vi "VibSystem3Signals.vi"(8 "sampling info":cluster{"Fs":dbl, "#s":dbl}={"Fs"=10000.0, "#s"=10000.0} {"Fs" format="%.2p"}, 9 "Temperature Channels Voltage In":dbl[](array[numeric]), 10 "Frequency":dbl, 11 "Constant Amplitudes?":bool) -> (1 "Temperature Channels Voltage Out":dbl[](array[numeric]), 3 "Signals":waveform(dbl)[](array[waveform]))   [LabVIEW 2017]
uses:
  <vilib>/measure/NI_MABase.lvlib
panel:
  out "Waveform Graph":waveform(dbl)[](graph)
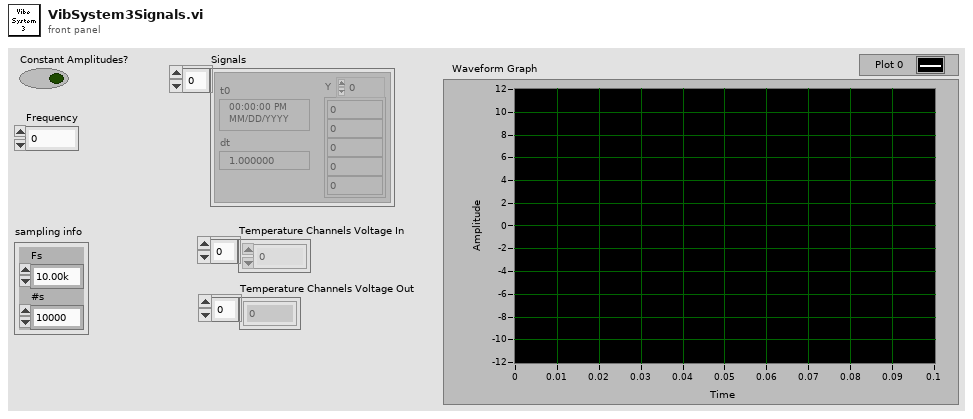
[diagram p1: front panel]
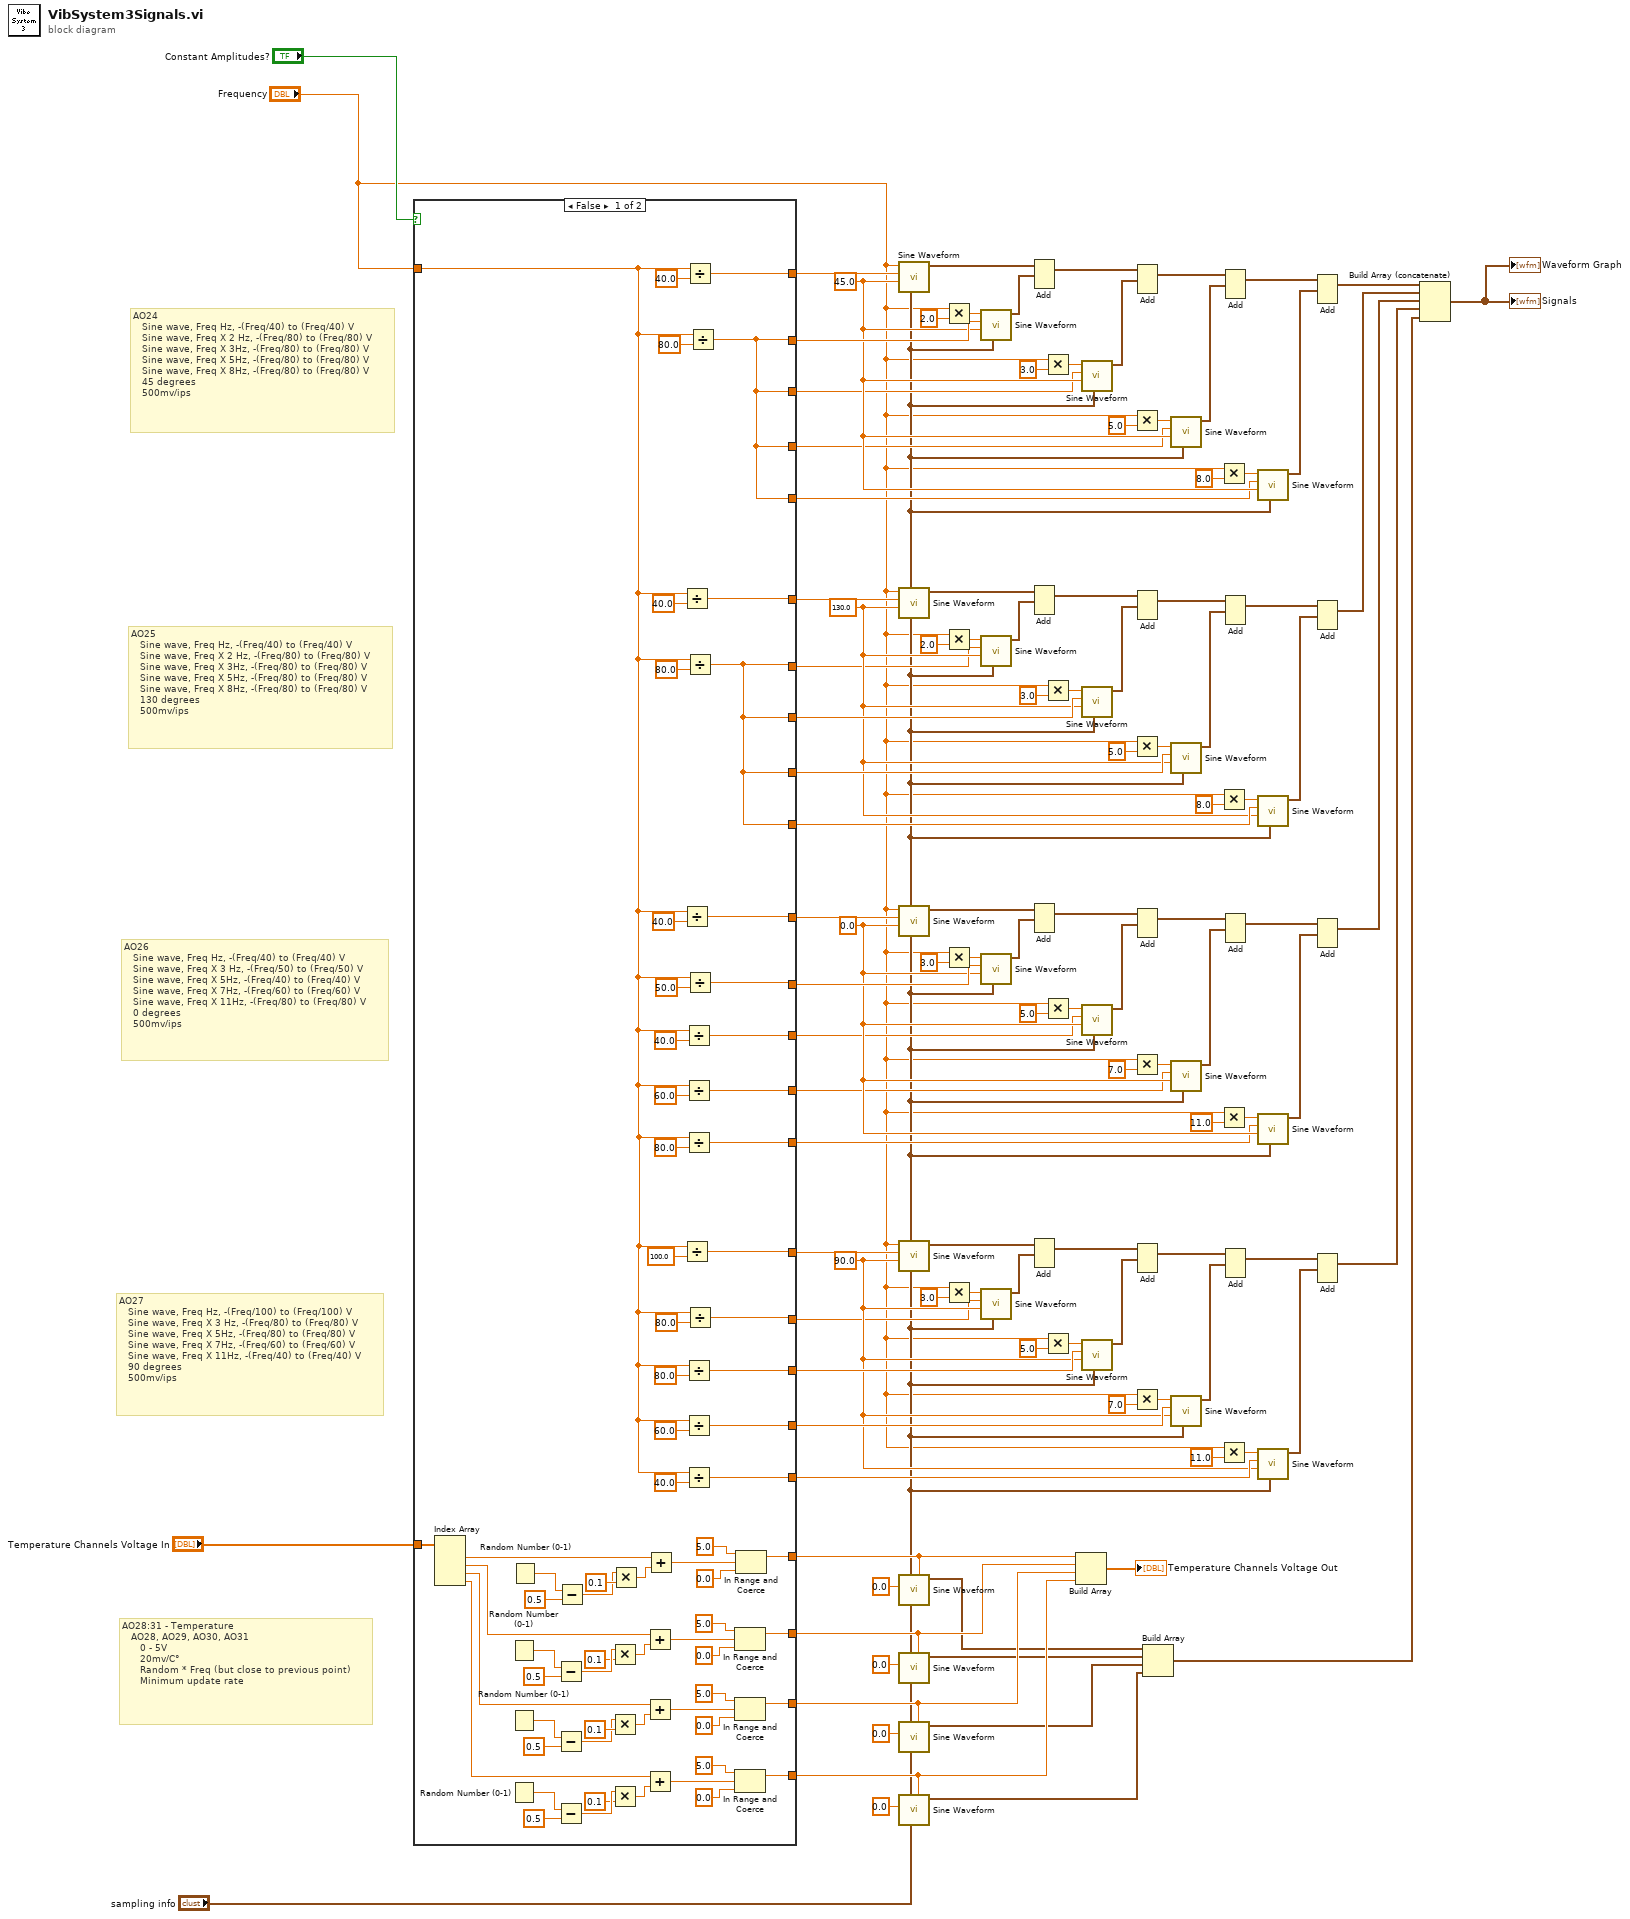
[diagram p0: block diagram]
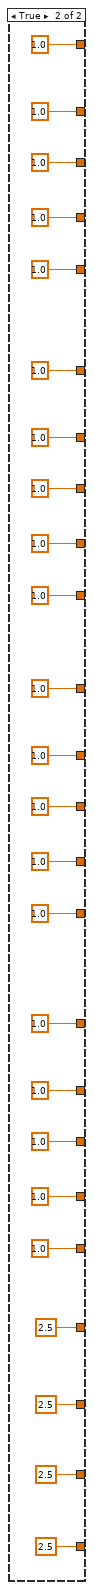
[diagram p2: hidden frame]
diagram:
  w16 = 90.0 ("phase")
  w36 = 0.0 ("phase")
  w74 = 130.0 ("phase")
  w97 = 45.0 ("phase")
  # "AO28:31 - Temperature\n   AO28, AO29, AO30, AO31\n      0 - 5V\n      20mv/C°\n      Random * Freq (but close to previous point)\n      Minimum update rate"
  # "AO27\n   Sine wave, Freq Hz, -(Freq/100) to (Freq/100) V\n   Sine wave, Freq X 3 Hz, -(Freq/80) to (Freq/80) V\n   Sine wave, Freq X 5Hz, -(Freq/80) to (Freq/80) V\n   Sine wave, Freq X 7Hz, -(Freq/60) to (Freq/60) V\n   Sine wave, Freq X 11Hz, -(Freq/40) to (Freq/40) V\n   90 degrees\n   500mv/ips"
  # "AO26\n   Sine wave, Freq Hz, -(Freq/40) to (Freq/40) V\n   Sine wave, Freq X 3 Hz, -(Freq/50) to (Freq/50) V\n   Sine wave, Freq X 5Hz, -(Freq/40) to (Freq/40) V\n   Sine wave, Freq X 7Hz, -(Freq/60) to (Freq/60) V\n   Sine wave, Freq X 11Hz, -(Freq/80) to (Freq/80) V\n   0 degrees\n   500mv/ips"
  # "AO25\n   Sine wave, Freq Hz, -(Freq/40) to (Freq/40) V\n   Sine wave, Freq X 2 Hz, -(Freq/80) to (Freq/80) V\n   Sine wave, Freq X 3Hz, -(Freq/80) to (Freq/80) V\n   Sine wave, Freq X 5Hz, -(Freq/80) to (Freq/80) V\n   Sine wave, Freq X 8Hz, -(Freq/80) to (Freq/80) V\n   130 degrees\n   500mv/ips"
  # "AO24\n   Sine wave, Freq Hz, -(Freq/40) to (Freq/40) V\n   Sine wave, Freq X 2 Hz, -(Freq/80) to (Freq/80) V\n   Sine wave, Freq X 3Hz, -(Freq/80) to (Freq/80) V\n   Sine wave, Freq X 5Hz, -(Freq/80) to (Freq/80) V\n   Sine wave, Freq X 8Hz, -(Freq/80) to (Freq/80) V\n   45 degrees\n   500mv/ips"
  n1 = case shown="False" "Constant Amplitudes?" {
    tunnel: [w180 1.0] -> w109
    tunnel: [w169 1.0] -> w110
    tunnel: "Frequency" -> [w112 _]
    tunnel: [w177 2.5 ("upper limit")] -> w85
    tunnel: [w169 1.0] -> w96
    tunnel: [w169 1.0] -> w88
    tunnel: [w169 1.0] -> w87
    tunnel: "Temperature Channels Voltage In" -> [w144 _]
    tunnel: [w139 2.5 ("upper limit")] -> w57
    tunnel: [w138 2.5 ("upper limit")] -> w56
    tunnel: [w137 2.5 ("upper limit")] -> w55
    tunnel: [w134 1.0] -> w63
    tunnel: [w133 1.0] -> w62
    tunnel: [w133 1.0] -> w75
    tunnel: [w133 1.0] -> w82
    tunnel: [w133 1.0] -> w83
    tunnel: [w132 1.0] -> w47
    tunnel: [w123 1.0] -> w48
    tunnel: [w124 1.0] -> w35
    tunnel: [w125 1.0] -> w28
    tunnel: [w126 1.0] -> w27
    tunnel: [w113 1.0] -> w5
    tunnel: [w122 1.0] -> w4
    tunnel: [w121 1.0] -> w17
    tunnel: [w120 1.0] -> w24
    tunnel: [w119 1.0] -> w25
    frame False {
      n2 = Index Array(array=w144) -> (element #1=w143:dbl, element #2=w142:dbl, element #3=w141:dbl, element #4=w140:dbl)  [unwired: 4 in]
      n3 = Random Number (0-1)() -> (number: 0 to 1=w164:dbl)
      n4 = Random Number (0-1)() -> (number: 0 to 1=w157:dbl)
      n5 = Random Number (0-1)() -> (number: 0 to 1=w148:dbl)
      n6 = Random Number (0-1)() -> (number: 0 to 1=w175:dbl)
      n7 = Subtract(x=w164, y=0.5) -> (x-y=w166:dbl)
      n8 = Subtract(x=w157, y=0.5) -> (x-y=w155:dbl)
      n9 = Subtract(x=w148, y=0.5) -> (x-y=w150:dbl)
      n10 = Subtract(x=w175, y=0.5) -> (x-y=w173:dbl)
      n11 = Multiply(x=w166, y=0.1) -> (x*y=w167:dbl)
      n12 = Multiply(x=w155, y=0.1) -> (x*y=w154:dbl)
      n13 = Multiply(x=w150, y=0.1) -> (x*y=w151:dbl)
      n14 = Multiply(x=w173, y=0.1) -> (x*y=w172:dbl)
      n15 = Add(x=w142, y=w167) -> (x+y=w168:dbl)
      n16 = Add(x=w141, y=w154) -> (x+y=w153:dbl)
      n17 = Add(x=w140, y=w151) -> (x+y=w152:dbl)
      n18 = Add(x=w143, y=w172) -> (x+y=w171:dbl)
      n19 = Divide(x=w112, y=40.0) -> (x/y=w134:dbl)
      n20 = Divide(x=w112, y=40.0) -> (x/y=w132:dbl)
      n21 = Divide(x=w112, y=100.0) -> (x/y=w113:dbl)
      n22 = Divide(x=w112, y=40.0) -> (x/y=w124:dbl)
      n23 = Divide(x=w112, y=60.0) -> (x/y=w125:dbl)
      n24 = Divide(x=w112, y=80.0) -> (x/y=w126:dbl)
      n25 = Divide(x=w112, y=80.0) -> (x/y=w121:dbl)
      n26 = Divide(x=w112, y=60.0) -> (x/y=w120:dbl)
      n27 = Divide(x=w112, y=40.0) -> (x/y=w119:dbl)
      n28 = Divide(x=w112, y=40.0) -> (x/y=w180:dbl)
      n29 = Divide(x=w112, y=80.0) -> (x/y=w133:dbl)
      n30 = Divide(x=w112, y=50.0) -> (x/y=w123:dbl)
      n31 = Divide(x=w112, y=80.0) -> (x/y=w122:dbl)
      n32 = Divide(x=w112, y=80.0) -> (x/y=w169:dbl)
      n33 = In Range and Coerce(upper limit=5.0, x=w168, lower limit=0.0) -> (coerced(x)=w139:dbl)  [unwired: 1 out]
      n34 = In Range and Coerce(upper limit=5.0, x=w153, lower limit=0.0) -> (coerced(x)=w138:dbl)  [unwired: 1 out]
      n35 = In Range and Coerce(upper limit=5.0, x=w152, lower limit=0.0) -> (coerced(x)=w137:dbl)  [unwired: 1 out]
      n36 = In Range and Coerce(upper limit=5.0, x=w171, lower limit=0.0) -> (coerced(x)=w177:dbl)  [unwired: 1 out]
    }
    frame True {
    }
  }
  n37 = call <vilib>:"Sine Waveform.vi"("sampling info"="sampling info", "phase"=w97, "amplitude"=w109, "frequency"="Frequency") -> ("signal out"=w107:waveform(dbl))  [unwired: 6 in, 1 out]
  n38 = call <vilib>:"Sine Waveform.vi"("sampling info"="sampling info", "phase"=w74, "amplitude"=w63, "frequency"="Frequency") -> ("signal out"=w64:waveform(dbl))  [unwired: 6 in, 1 out]
  n39 = call <vilib>:"Sine Waveform.vi"("sampling info"="sampling info", "phase"=w36, "amplitude"=w47, "frequency"="Frequency") -> ("signal out"=w46:waveform(dbl))  [unwired: 6 in, 1 out]
  n40 = call <vilib>:"Sine Waveform.vi"("sampling info"="sampling info", "phase"=w16, "amplitude"=w5, "frequency"="Frequency") -> ("signal out"=w6:waveform(dbl))  [unwired: 6 in, 1 out]
  n41 = call <vilib>:"Sine Waveform.vi"("offset"=w85, "sampling info"="sampling info", "amplitude"=0.0) -> ("signal out"=w54:waveform(dbl))  [unwired: 7 in, 1 out]
  n42 = call <vilib>:"Sine Waveform.vi"("offset"=w57, "sampling info"="sampling info", "amplitude"=0.0) -> ("signal out"=w53:waveform(dbl))  [unwired: 7 in, 1 out]
  n43 = call <vilib>:"Sine Waveform.vi"("offset"=w56, "sampling info"="sampling info", "amplitude"=0.0) -> ("signal out"=w52:waveform(dbl))  [unwired: 7 in, 1 out]
  n44 = call <vilib>:"Sine Waveform.vi"("offset"=w55, "sampling info"="sampling info", "amplitude"=0.0) -> ("signal out"=w51:waveform(dbl))  [unwired: 7 in, 1 out]
  n45 = Multiply(x="Frequency", y=2.0) -> (x*y=w104:dbl)
  n46 = Multiply(x="Frequency", y=2.0) -> (x*y=w67:dbl)
  n47 = Multiply(x="Frequency", y=3.0) -> (x*y=w43:dbl)
  n48 = Multiply(x="Frequency", y=3.0) -> (x*y=w9:dbl)
  n49 = call <vilib>:"Sine Waveform.vi"("sampling info"="sampling info", "phase"=w97, "amplitude"=w110, "frequency"=w104) -> ("signal out"=w106:waveform(dbl))  [unwired: 6 in, 1 out]
  n50 = call <vilib>:"Sine Waveform.vi"("sampling info"="sampling info", "phase"=w74, "amplitude"=w62, "frequency"=w67) -> ("signal out"=w65:waveform(dbl))  [unwired: 6 in, 1 out]
  n51 = call <vilib>:"Sine Waveform.vi"("sampling info"="sampling info", "phase"=w36, "amplitude"=w48, "frequency"=w43) -> ("signal out"=w45:waveform(dbl))  [unwired: 6 in, 1 out]
  n52 = call <vilib>:"Sine Waveform.vi"("sampling info"="sampling info", "phase"=w16, "amplitude"=w4, "frequency"=w9) -> ("signal out"=w7:waveform(dbl))  [unwired: 6 in, 1 out]
  n53 = Add(1:w106, 2:w107) -> (0:w95:waveform(dbl))  [unwired: 1 in, 1 out]
  n54 = Add(1:w65, 2:w64) -> (0:w76:waveform(dbl))  [unwired: 1 in, 1 out]
  n55 = Add(1:w45, 2:w46) -> (0:w34:waveform(dbl))  [unwired: 1 in, 1 out]
  n56 = Add(1:w7, 2:w6) -> (0:w18:waveform(dbl))  [unwired: 1 in, 1 out]
  n57 = Multiply(x="Frequency", y=3.0) -> (x*y=w103:dbl)
  n58 = Multiply(x="Frequency", y=3.0) -> (x*y=w68:dbl)
  n59 = Multiply(x="Frequency", y=5.0) -> (x*y=w42:dbl)
  n60 = Multiply(x="Frequency", y=5.0) -> (x*y=w10:dbl)
  n61 = Build Array(w85, w57, w56, w55) -> (→"Temperature Channels Voltage Out":dbl[])
  n62 = call <vilib>:"Sine Waveform.vi"("sampling info"="sampling info", "phase"=w97, "amplitude"=w96, "frequency"=w103) -> ("signal out"=w94:waveform(dbl))  [unwired: 6 in, 1 out]
  n63 = call <vilib>:"Sine Waveform.vi"("sampling info"="sampling info", "phase"=w74, "amplitude"=w75, "frequency"=w68) -> ("signal out"=w77:waveform(dbl))  [unwired: 6 in, 1 out]
  n64 = call <vilib>:"Sine Waveform.vi"("sampling info"="sampling info", "phase"=w36, "amplitude"=w35, "frequency"=w42) -> ("signal out"=w33:waveform(dbl))  [unwired: 6 in, 1 out]
  n65 = call <vilib>:"Sine Waveform.vi"("sampling info"="sampling info", "phase"=w16, "amplitude"=w17, "frequency"=w10) -> ("signal out"=w19:waveform(dbl))  [unwired: 6 in, 1 out]
  n66 = Add(1:w94, 2:w95) -> (0:w93:waveform(dbl))  [unwired: 1 in, 1 out]
  n67 = Multiply(x="Frequency", y=5.0) -> (x*y=w100:dbl)
  n68 = Add(1:w77, 2:w76) -> (0:w78:waveform(dbl))  [unwired: 1 in, 1 out]
  n69 = Multiply(x="Frequency", y=5.0) -> (x*y=w71:dbl)
  n70 = Add(1:w33, 2:w34) -> (0:w32:waveform(dbl))  [unwired: 1 in, 1 out]
  n71 = Multiply(x="Frequency", y=7.0) -> (x*y=w39:dbl)
  n72 = Add(1:w19, 2:w18) -> (0:w20:waveform(dbl))  [unwired: 1 in, 1 out]
  n73 = Multiply(x="Frequency", y=7.0) -> (x*y=w13:dbl)
  n74 = Build Array(w54, w53, w52, w51) -> (w50:waveform(dbl)[])
  n75 = call <vilib>:"Sine Waveform.vi"("sampling info"="sampling info", "phase"=w97, "amplitude"=w88, "frequency"=w100) -> ("signal out"=w92:waveform(dbl))  [unwired: 6 in, 1 out]
  n76 = call <vilib>:"Sine Waveform.vi"("sampling info"="sampling info", "phase"=w74, "amplitude"=w82, "frequency"=w71) -> ("signal out"=w79:waveform(dbl))  [unwired: 6 in, 1 out]
  n77 = call <vilib>:"Sine Waveform.vi"("sampling info"="sampling info", "phase"=w36, "amplitude"=w28, "frequency"=w39) -> ("signal out"=w31:waveform(dbl))  [unwired: 6 in, 1 out]
  n78 = call <vilib>:"Sine Waveform.vi"("sampling info"="sampling info", "phase"=w16, "amplitude"=w24, "frequency"=w13) -> ("signal out"=w21:waveform(dbl))  [unwired: 6 in, 1 out]
  n79 = Multiply(x="Frequency", y=8.0) -> (x*y=w99:dbl)
  n80 = Multiply(x="Frequency", y=8.0) -> (x*y=w72:dbl)
  n81 = Multiply(x="Frequency", y=11.0) -> (x*y=w38:dbl)
  n82 = Multiply(x="Frequency", y=11.0) -> (x*y=w14:dbl)
  n83 = Add(1:w92, 2:w93) -> (0:w91:waveform(dbl))  [unwired: 1 in, 1 out]
  n84 = Add(1:w79, 2:w78) -> (0:w80:waveform(dbl))  [unwired: 1 in, 1 out]
  n85 = Add(1:w31, 2:w32) -> (0:w30:waveform(dbl))  [unwired: 1 in, 1 out]
  n86 = Add(1:w21, 2:w20) -> (0:w22:waveform(dbl))  [unwired: 1 in, 1 out]
  n87 = call <vilib>:"Sine Waveform.vi"("sampling info"="sampling info", "phase"=w97, "amplitude"=w87, "frequency"=w99) -> ("signal out"=w90:waveform(dbl))  [unwired: 6 in, 1 out]
  n88 = call <vilib>:"Sine Waveform.vi"("sampling info"="sampling info", "phase"=w74, "amplitude"=w83, "frequency"=w72) -> ("signal out"=w81:waveform(dbl))  [unwired: 6 in, 1 out]
  n89 = call <vilib>:"Sine Waveform.vi"("sampling info"="sampling info", "phase"=w36, "amplitude"=w27, "frequency"=w38) -> ("signal out"=w29:waveform(dbl))  [unwired: 6 in, 1 out]
  n90 = call <vilib>:"Sine Waveform.vi"("sampling info"="sampling info", "phase"=w16, "amplitude"=w25, "frequency"=w14) -> ("signal out"=w23:waveform(dbl))  [unwired: 6 in, 1 out]
  n91 = Add(1:w90, 2:w91) -> (0:w89:waveform(dbl))  [unwired: 1 in, 1 out]
  n92 = Add(1:w81, 2:w80) -> (0:w49:waveform(dbl))  [unwired: 1 in, 1 out]
  n93 = Add(1:w29, 2:w30) -> (0:w26:waveform(dbl))  [unwired: 1 in, 1 out]
  n94 = Add(1:w23, 2:w22) -> (0:w1:waveform(dbl))  [unwired: 1 in, 1 out]
  n95 = Build Array (concatenate)(w89, w49, w26, w1, w50) -> (→"Signals" →"Waveform Graph":waveform(dbl)[])
